vi "Pre Launch Init.vi"(11 "Actor_Scope in":refnum<class "Actor_Scope.lvclass">) -> (0 "error out":errorcluster, 3 "Actor_Scope out":refnum<class "Actor_Scope.lvclass">)   [LabVIEW 2020, in "Actor_Scope.lvlib" / "Actor_Scope.lvclass"]
doc: "(<B>Filename</B>: Actor Framework.lvlib:Actor.lvclass:Pre Launch Init.vi)\n\nDefines behavior that occurs after the Launch Nested Actor method is invoked but before the actor's Actor Core method begins running.\n\nBy default, this method does nothing. A descendant class may override it to define behavior."
uses:
  Actor_Scope.lvclass
  C:/Program Files/National Instruments/LabVIEW 2020/vi.lib/ActorFramework/Actor/Actor.lvclass
  <vilib>/ActorFramework/Actor/Actor.lvclass/Actor.ctl
  Actor_Scope.lvclass/Actor_Scope.ctl
  Scope_Event.ctl
  <vilib>/ActorFramework/Actor/Actor.lvclass
  <instrlib>/Agilent 8000 Series/Agilent 8000 Series.lvlib
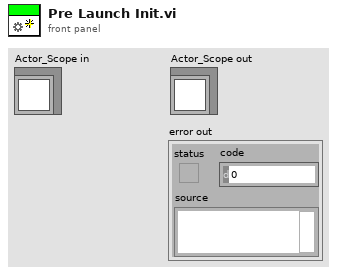
[diagram p1: front panel]
types:
  T1 = typedef "Actor_Scope.lvlib/Actor_Scope.lvclass/Scope_Event.ctl" = enum16{"General Event", "Inited", "Error", "Wfm Acq Complete"}
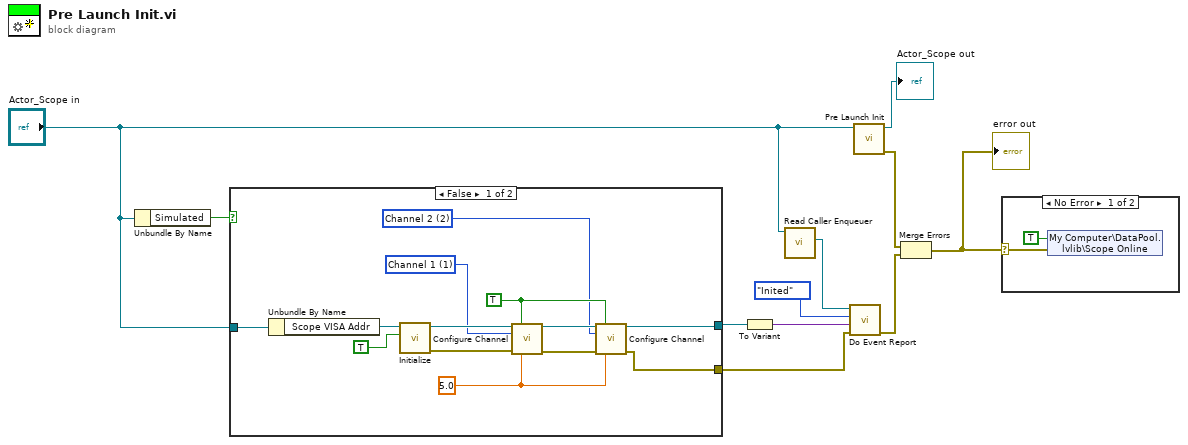
[diagram p0: block diagram]
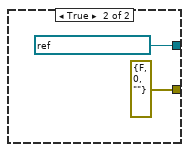
[diagram p3: hidden frame]
diagram:
  n1 = Unbundle By Name("Actor_Scope in") -> ("Simulated"=w9:bool)
  n2 = case shown="False" w9 {
    tunnel: "Actor_Scope in" -> [w24 _]
    tunnel: [w13 refnum<visa-resource-name> "Simulated Scope" ("VISA resource name out")] -> w10
    tunnel: [w12 errorcluster {"status"=FALSE, "code"=0, "source"=""} ("error out")] -> w3
    frame False {
      w14 = 5.0 ("Vertical Range (2.0 V)")
      w15 = 2 items=["Channel 1"=1, "Channel 2"=2, "Channel 3"=3, "Channel 4"=4] ("Channel (1: Channel 1)")
      w16 = 1 items=["Channel 1"=1, "Channel 2"=2, "Channel 3"=3, "Channel 4"=4] ("Channel (1: Channel 1)")
      w17 = TRUE ("Enable Channel (Enable)")
      n3 = Unbundle By Name(w24) -> ("Scope VISA Addr"=w23:refnum<visa-resource-name>)
      n4 = call <instrlib>:"Initialize.vi"("ID Query (True)"=TRUE, "VISA resource name"=w23) -> ("error out"=w20:errorcluster, "VISA resource name out"=w21:refnum<visa-resource-name>)  [unwired: 8 in]
      n5 = call <instrlib>:"Configure Channel.vi"("VISA resource name"=w21, "Enable Channel (Enable)"=w17, "Channel (1: Channel 1)"=w16, "error in (no error)"=w20, "Vertical Range (2.0 V)"=w14) -> ("VISA resource name out"=w19:refnum<visa-resource-name>, "error out"=w18:errorcluster)  [unwired: 9 in]
      n6 = call <instrlib>:"Configure Channel.vi"("VISA resource name"=w19, "Enable Channel (Enable)"=w17, "Channel (1: Channel 1)"=w15, "error in (no error)"=w18, "Vertical Range (2.0 V)"=w14) -> ("VISA resource name out"=w13:refnum<visa-resource-name>, "error out"=w12:errorcluster)  [unwired: 9 in]
    }
    frame True {
    }
  }
  n7 = To Variant(anything=w10) -> (Variant=w4:variant)
  n8 = call <vilib>:"Read Caller Enqueuer.vi"("Actor"="Actor_Scope in") -> ("Caller Enqueuer"=w5:refnum<class "Message Enqueuer.lvclass">)  [unwired: 10 in]
  n9 = call "Do Event Report.vi"("error in (no error)"=w3, "Event Data"=w4, "Scope Events"=Scope_Event."Inited", "Caller Enqueuer"=w5) -> ("error out"=w2:errorcluster)  [unwired: 6 in, 1 out]
  n10 = call-parent "Pre Launch Init.vi"("Actor in"="Actor_Scope in") -> ("error out"=w8:errorcluster, "Actor out"=→"Actor_Scope out":refnum<class "Actor_Scope.lvclass">)  [unwired: 9 in]
  n11 = Merge Errors(w8, w2) -> (w7:errorcluster)
  "error out" <- w7
  n12 = case shown="No Error" w7 {
    selector: w7 -> [w28 _]
    frame No Error {
      n13 = shared-variable "My Computer\\DataPool.lvlib\\Scope Online"(TRUE ("AFG Online"), error in=w28) -> ()  [unwired: 1 out]
    }
    frame Error {
    }
  }
